vi "MEMR-Process Database.vi"() -> ()   [LabVIEW 2015]
uses:
  <vilib>/Analysis/NI_AALBase.lvlib
panel:
  out "Histogram Graph":T1(graph)={"X Values"=[-47.631112187359534, -42.893336562078595, -38.155560936797656, -33.41778531151672, -28.68000968623578, -23.942234060954842, -19.204458435673907, -14.466682810392967, -9.72890718511203, -4.991131559831092, -0.2533559345501544, 4.484419690730784, 9.222195316011721, 13.959970941292658, 18.697746566573596, 23.435522191854535, 28.17329781713547, 32.91107344241641, 37.64884906769735, 42.38662469297829], "Histogram: h(x)"=[2, 3, 2, 1, 2, 3, 5, 11, 7, 26, 28, 31, 12, 21, 13, 5, 5, 2, 1, 1]}
  in  "Analysis":T2={"Mode"=enum."at max gain", "T(ms) re peak"=2.0, "Fmin (Hz)"=800.0, "Fmax (Hz)"=3200.0, "Window"=enum."Hamming", "Resol (Hz)"=100.0, "Width (Hz)"=600.0, "Width (Hz) 2"=600.0}
  out "XY Graph":cluster{dbl[], dbl[]}[](graph)=[{[65.0, 70.0, 75.0, 70.0, 70.0, 65.0, 75.0, 70.0, 70.0, 70.0, 70.0, 70.0, 75.0, 85.0, 80.0, 80.0, 70.0, 75.0, 80.0, 80.0, 75.0, 65.0, 90.0, 90.0, 70.0, 75.0, 75.0, 65.0, 70.0, 70.0, 80.0, 75.0, 85.0, 80.0, 85.0, 80.0, 70.0, 65.0, 85.0, 80.0, 65.0, 75.0, 80.0, 75.0, 80.0, nan, 60.0, 60.0, 60.0, nan, 85.0, 80.0, 70.0, 70.0, 75.0, 85.0, 95.0, 75.0, 100.0, 85.0, 75.0, 90.0, 80.0, 75.0, 95.0, 90.0, 95.0, 90.0, 65.0, 75.0, nan, nan, 80.0, 80.0, 75.0, 90.0, 70.0, 85.0, 80.0, 50.0, 95.0, 90.0, 95.0, 85.0, 65.0, nan, 65.0, 75.0, 50.0, 65.0, 80.0, 80.0, 70.0, 90.0, 80.0, 70.0, 80.0, 75.0, 90.0, 85.0, 70.0, 70.0, 95.0, nan, 90.0, 80.0, 95.0, 100.0, 100.0, 100.0, 50.0, 85.0, 70.0, 50.0, 75.0, 75.0, 75.0, 75.0, 80.0, 85.0, 75.0, 75.0, 85.0, 70.0, 80.0, nan, 100.0, 85.0, 85.0, 80.0, 100.0, 75.0, 90.0, 85.0, 80.0, 75.0, 80.0, 75.0, 90.0, 90.0, 85.0, 75.0, 90.0, 90.0, 65.0, 85.0, 65.0, 65.0, 65.0, 85.0, 85.0, 90.0, nan, 85.0, 80.0, 75.0, 85.0, 80.0, 80.0, 75.0, 65.0, nan, 75.0, 70.0, 85.0, 75.0, 65.0, 75.0, 80.0, 75.0, 75.0, 50.0, 70.0, 80.0, 75.0, 70.0, 95.0, 85.0, 100.0, 90.0, 80.0, 80.0, 95.0, 90.0, 90.0, 50.0, 95.0, 95.0, 65.0, 75.0, 70.0, 70.0, 75.0, 80.0, 65.0, 65.0, 85.0, 60.0, 75.0, 70.0, 70.0, 75.0, 80.0, 80.0, 60.0, 85.0, 80.0, 75.0, 85.0, 80.0, 80.0, 80.0, 75.0, 75.0, nan, 80.0, 85.0, 80.0, 90.0, nan, 75.0, nan, 75.0, 80.0, 80.0, 70.0, nan, nan, 80.0, 50.0, 70.0, nan, 80.0, 70.0, 75.0, 60.0, 65.0, nan], [83.61038480664206, 88.90323491138284, nan, 76.6861342480343, 79.34245681049052, 66.14502666631483, 72.64039776246874, nan, 90.40140695048568, 73.59986593514996, 68.2285833975198, 68.95909577888109, 78.34029194041977, 66.40476363843403, nan, 88.4677553721679, 84.58576085004772, 62.13837967961564, 75.27817702322353, 71.94988571809287, 76.92571447237148, nan, 85.70082896210121, 87.89120704634068, 94.67191690824791, 79.80233146849612, 73.85409029034139, nan, 85.0, 93.55766432018085, 71.17769645171938, 85.4769276924145, nan, 84.75979569569505, 85.0, 85.52670684346738, 66.9788899682501, 69.20948606719492, 78.12781009882714, 79.19224304801239, 69.01017671276524, 67.64300936225919, 75.8043887454742, 73.85609821156797, 76.01253626857745, 85.0, 87.67149436103365, 66.75304409750719, 77.92784007393945, 82.44046631465581, 76.97482808652369, 78.44429598980619, 90.36011233515646, 57.49379196106444, 68.14676914537219, 78.66064680390217, nan, nan, nan, nan, 81.20509176100323, nan, 85.0, 70.33095954554724, 45.0, nan, 87.68722889473402, 85.25509994697506, 94.78893078630351, 77.75515257560767, 90.0, nan, nan, 94.8348417211292, 83.00419918222694, 93.18892634377539, 83.45013835841418, 72.03015940057925, 94.78202672029386, 79.7564120495189, 53.50224673653963, 85.84587239002288, 91.08548698295861, 46.25077363388457, 84.78546328663008, 91.01701177396114, 70.30568906673099, 78.99595778229026, 75.90995049601652, 85.02181316130722, 89.48615624550615, 81.1093912479705, 89.64413251768113, nan, 72.09675267675055, 81.72805574099463, 76.34503888270152, 75.67164645735843, 76.72561644593952, 54.108997651036915, 85.78378392899137, 78.47759249254159, 50.0, nan, nan, nan, 84.27014033057675, nan, 85.0, 89.83440652992289, 90.0, 63.3780833666432, 82.275627583266, 69.4041108088633, 77.55665508198922, 73.3088683958336, 86.90689069975696, 74.96703575207891, 82.37700129008836, 83.63890795813947, 72.19417062306756, 71.20730347534435, 90.95563139214721, 82.26302545197102, 59.757364077419076, 77.11292838155504, 87.08209177013414, nan, 80.0, 83.43169269612767, 53.73146823384199, 87.13006660761161, nan, 53.43379419404157, 80.01393285329306, 80.54156385472628, 80.21327744960064, 68.59887423802961, 70.0, nan, 82.77268093940407, 70.79201679725688, 88.65228346267106, 67.69603653315627, 70.0, 60.0, 90.0, 76.67991571420627, 80.0, 88.353883211932, 83.52892385361397, 70.0, 50.0, nan, 92.1153796896727, 77.80998882203835, nan, 89.76332680957675, 80.97331020337515, 72.83227440234356, 78.98506818754085, nan, 75.73931301525411, 85.0, 94.42464287719379, 84.08850701174643, nan, 75.35249373246242, 65.0, 90.0, 91.04866573115002, 80.90730659397525, 79.81740356491906, 85.0, 84.44661858514274, 90.48293650558534, 88.2586818731154, 77.00692996492972, nan, nan, 85.0, 83.56030129511086, 73.99166681322971, 75.0, 49.751203636703785, 43.722271947164565, 91.30805595730399, 65.0, nan, 75.09348869162191, 88.26860390703759, nan, 68.3141967304181, nan, 84.94480698741687, 87.85999618819487, 41.93345844004098, nan, nan, nan, nan, 90.0, 73.4554146040901, nan, 84.34738292000237, 68.43165488319733, 63.833644698525994, 91.47936652555856, 93.67058040834105, nan, nan, nan, 73.87445771753136, 78.30397650963862, 79.38295699025869, 93.49248113271616, 88.06829172475629, nan, nan, nan, 70.0, nan, 80.0, nan, 86.30759278580638, nan, 60.0, nan, 81.01066592260895, 94.75551250561875, nan, 91.62181131893622, 67.40528394856256, 72.50990150751193, 90.0, 94.1375552879297, 90.94631112233287, 74.72565053329737]}, ...(2 in all)]
  out "Progress":string="238/238"
  in  "Database":path=path "D:/Data/HHL/MEMR/database MEMR.csv"
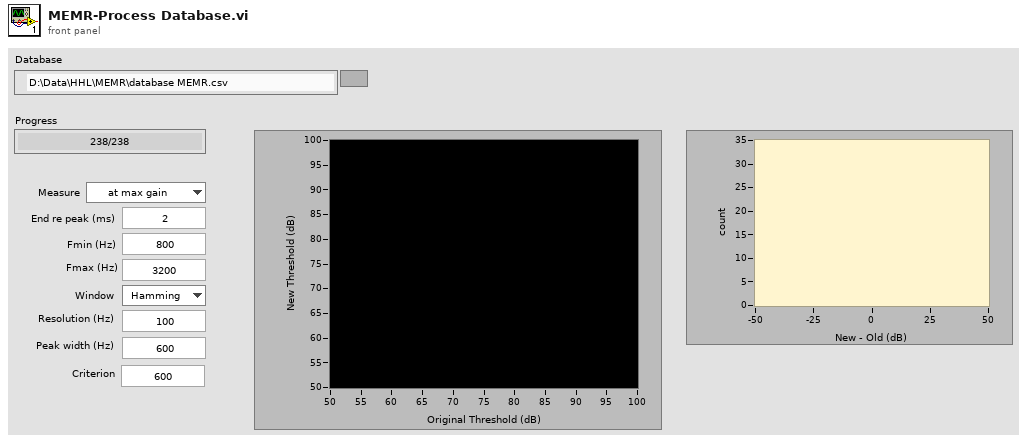
[diagram p1: front panel]
types:
  T1 = cluster{"X Values":dbl[], "Histogram: h(x)":i32[]}
  T2 = cluster{"Mode":enum16{"at max mag", "at max gain", "over window", "optimize"}, "T(ms) re peak":dbl, "Fmin (Hz)":dbl, "Fmax (Hz)":dbl, "Window":enum16{"None", "Hanning", "Hamming"}, "Resol (Hz)":dbl, "Width (Hz)":dbl, "Width (Hz) 2":dbl}
  T3 = enum16{"at max mag", "at max gain", "over window", "optimize"}
  T4 = cluster{"ID":i32, "Ear":string, "Run":i32[], "Original":dbl, "Paths":path[], "Threshold":dbl, "Strength":dbl}
  T5 = typedef "PDF-Catalog.ctl" = cluster{"report":refnum<class "PDF Report Class.lvclass">, "rows":i32, "cols":i32, "border":dbl, "width":dbl, "height":dbl, "next":i32}
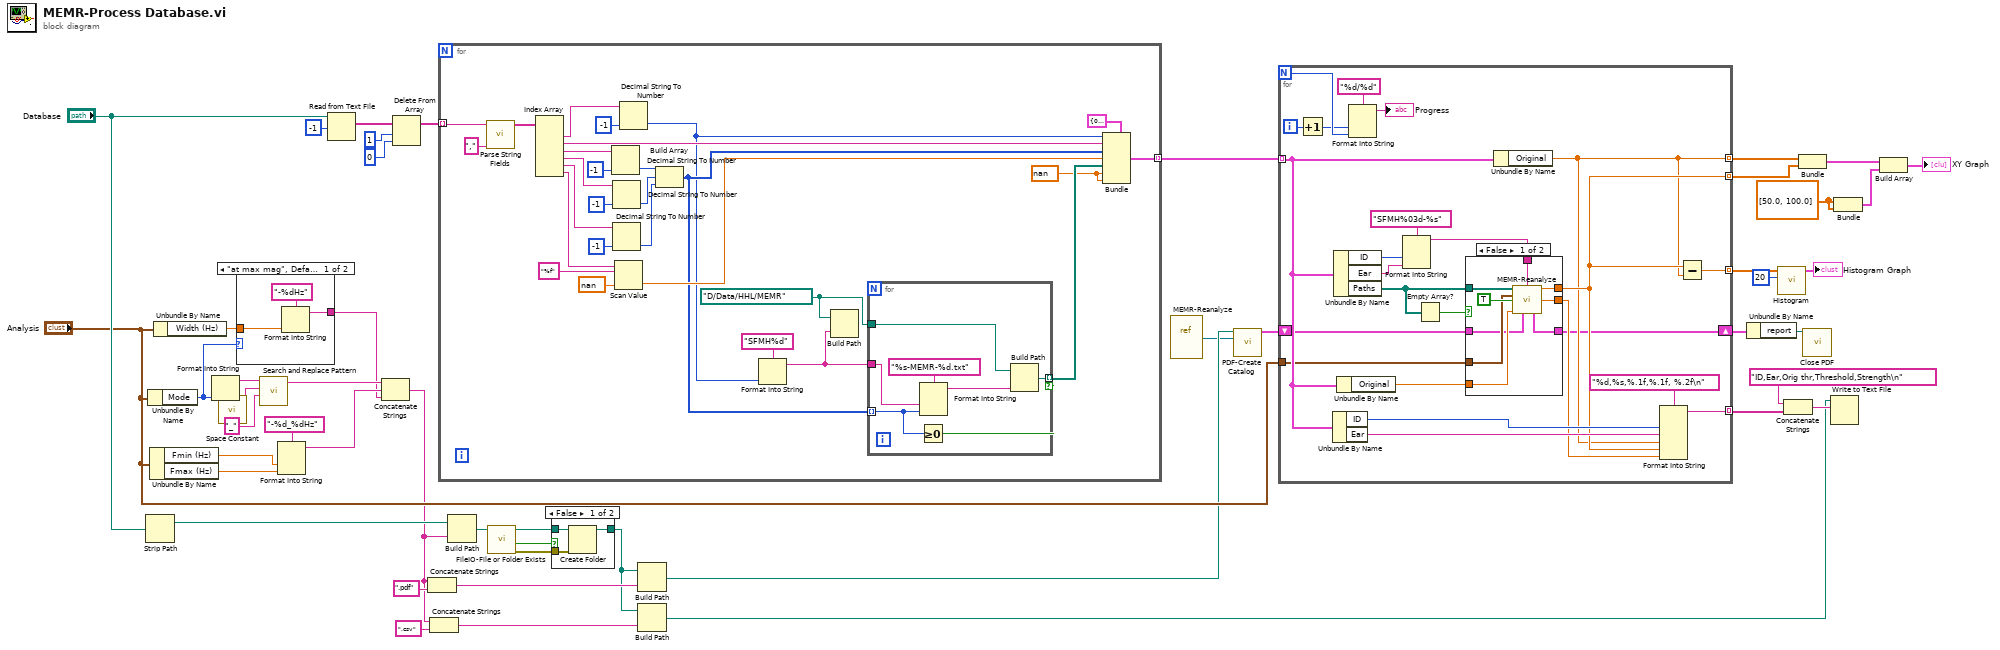
[diagram p0: block diagram]
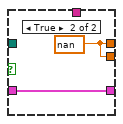
[diagram p4: hidden frame]
diagram:
  w40 = dbl[] [50.0, 100.0]
  n1 = Strip Path(path="Database") -> (stripped path=w19:path)  [unwired: 1 out]
  n2 = Unbundle By Name("Analysis") -> ("Mode"=w25:T3)
  n3 = Unbundle By Name("Analysis") -> ("Fmin (Hz)"=w27:dbl, "Fmax (Hz)"=w26:dbl)
  n4 = Unbundle By Name("Analysis") -> ("Width (Hz)"=w23:dbl)
  n5 = Format Into String(w25) -> (resulting string=w31:string)  [unwired: 3 in, 1 out]
  n6 = call <vilib>:"Space Constant.vi"() -> ("String"=w30:string)
  n7 = case shown="\"at max mag\", Default" w25 {
    tunnel: w23 -> [w51 _]
    tunnel: [w49 _] -> w20
    frame "at max mag", Default {
      n8 = Format Into String(format string="-%dHz", w51) -> (resulting string=w49:string)  [unwired: 2 in, 1 out]
    }
    frame "over window" {
    }
  }
  n9 = call <vilib>:"Search and Replace Pattern.vi"("string"=w31, "regular expression (\"\")"=w30, "replace string (\"\")"="_" ("replace string (\"\")")) -> ("result string"=w22:string)  [unwired: 2 in, 1 out]
  n10 = Format Into String(format string="-%d_%dHz", w27, w26) -> (resulting string=w21:string)  [unwired: 2 in, 1 out]
  n11 = Read from Text File(file (use dialog)="Database", count=-1) -> (text=w47:string[])  [unwired: 2 in, 3 out]
  n12 = Concatenate Strings(w22, w21, w20) -> (w7:string)
  n13 = Delete From Array(array=w47, length=1, index=0) -> (array with subset deleted=w44:string[])  [unwired: 1 out]
  n14 = Concatenate Strings(w7, ".pdf" ("string")) -> (w9:string)
  n15 = Concatenate Strings(w7, ".csv" ("string")) -> (w17:string)
  n16 = for {
    tunnel: w44 -> [w79] mode=indexing
    tunnel: [w63] -> w37 mode=indexing
    w53 = nan
    w52 = path "D:/Data/HHL/MEMR"
    n17 = call "Parse String Fields.vi"("Separator"=",", "String"=w79) -> ("Fields"=w77:string[])  [unwired: 8 in, 1 out]
    n18 = Index Array(array=w77) -> (element #1=w55:string, element #2=w58:string, element #3=w76:string, element #4=w72:string, element #5=w71:string, element #6=w70:string)  [unwired: 6 in]
    n19 = Decimal String To Number(string=w76, default (0L)=-1 ("default (0 I32)")) -> (number=w67:i32)  [unwired: 1 in, 1 out]
    n20 = Decimal String To Number(string=w72, default (0L)=-1 ("default (0 I32)")) -> (number=w66:i32)  [unwired: 1 in, 1 out]
    n21 = Decimal String To Number(string=w71, default (0L)=-1 ("default (0 I32)")) -> (number=w65:i32)  [unwired: 1 in, 1 out]
    n22 = Scan Value(string=w70, format string="%f", default (0 dbl)=nan) -> (value=w64:dbl)  [unwired: 1 out]
    n23 = Decimal String To Number(string=w55, default (0L)=-1 ("default (0 I32)")) -> (number=w54:i32)  [unwired: 1 in, 1 out]
    n24 = Build Array(w67, w66, w65) -> (w59:i32[])
    n25 = Format Into String(format string="SFMH%d", w54) -> (resulting string=w60:string)  [unwired: 2 in, 1 out]
    n26 = Build Path(base path=w52, name or relative path=w60) -> ()  [unwired: 1 out]
    n27 = for {
      tunnel: w52 -> [w83]
      tunnel: w59 -> [w81] mode=indexing
      tunnel: w60 -> [w85]
      tunnel: [w82] -> w57 mode=indexing if=w80
      n28 = Greater Or Equal To 0?(x=w81) -> (x >= 0?=w80:bool)
      n29 = Format Into String(format string="%s-MEMR-%d.txt", w85, w81) -> (resulting string=w84:string)  [unwired: 2 in, 1 out]
      n30 = Build Path(base path=w83, name or relative path=w84) -> (appended path=w82:path)
    }
    n31 = Bundle(cluster=T4 {"ID"=0, "Ear"="R", "Run"=[19, 20, 21], "Original"=65.0, "Paths"=[], "Threshold"=65.0, "Strength"=nan}, "ID"=w54, "Ear"=w58, "Run"=w59, "Original"=w64, "Paths"=w57, "Threshold"=w53, "Strength"=w53) -> (w63:T4)
  }
  n32 = Build Path(base path=w19, name or relative path=w7) -> (appended path=w8:path)
  n33 = call "FileIO-File or Folder Exists.vi"("path"=w8) -> ("error out"=w13:errorcluster, "Exists?"=w11:bool, "dup path"=w12:path)  [unwired: 7 in, 1 out]
  n34 = case shown="False" w11 {
    tunnel: [w89 w90] -> w3
    tunnel: w13 -> [w88 _]
    tunnel: w12 -> [w87 w90]
    frame False {
      n35 = Create Folder(path (use dialog)=w87, error in=w88) -> (created path=w89:path)  [unwired: 1 in, 2 out]
    }
    frame True {
    }
  }
  n36 = Build Path(base path=w3, name or relative path=w9) -> (appended path=w6:path)
  n37 = Build Path(base path=w3, name or relative path=w17) -> (appended path=w14:path)
  n38 = vi-ref "MEMR-Reanalyze.vi"() -> (w1:refnum<vi>)
  n39 = call "PDF-Create Catalog.vi"("PDF Path"=w6, "VI"=w1) -> ("catalog"=w5:T5)  [unwired: 12 in, 1 out]
  n40 = for {
    N -> [w109]
    tunnel: w37 -> [w102] mode=indexing
    tunnel: [w95] -> w43 mode=indexing
    tunnel: [w96] -> w42 mode=indexing
    tunnel: [w98] -> w36 mode=indexing
    tunnel: [w97] -> w35 mode=indexing
    tunnel: "Analysis" -> [w94]
    shift-right: [w92] -> w4
    shift-left: w5 -> [w93]
    i -> [w110]
    n41 = Increment(x=w110) -> (x+1=w107:i32)
    n42 = Unbundle By Name(w102) -> ("ID"=w101:i32, "Ear"=w100:string)
    n43 = Unbundle By Name(w102) -> ("ID"=w113:i32, "Ear"=w112:string, "Paths"=w106:path[])
    n44 = Unbundle By Name(w102) -> ("Original"=w104:dbl)
    n45 = Format Into String(format string="%d/%d", w107, w109) -> (resulting string=→"Progress":string)  [unwired: 2 in, 1 out]
    n46 = Format Into String(format string="SFMH%03d-%s", w113, w112) -> (resulting string=w91:string)  [unwired: 2 in, 1 out]
    n47 = Empty Array?(array=w106) -> (empty?=w105:bool)
    n48 = case shown="False" w105 {
      tunnel: [w122 w125] -> w96
      tunnel: w106 -> [w121 _]
      tunnel: w104 -> [w120 _]
      tunnel: [w119 w125] -> w99
      tunnel: w94 -> [w118 _]
      tunnel: w93 -> [w117 w124]
      tunnel: [w116 w124] -> w92
      tunnel: w91 -> [w115 _]
      frame False {
        n49 = call "MEMR-Reanalyze.vi"("Path"=w121, "Caption"=w115, "Threshold"=w118, "Plot?"=TRUE, "Original"=w120, "catalog in"=w117) -> ("Threshold"=w122:dbl, "Strength"=w119:dbl, "catalog out"=w116:T5)  [unwired: 7 in]
      }
      frame True {
        w125 = nan ("Threshold")
      }
    }
    n50 = Unbundle By Name(w102) -> ("Original"=w95:dbl)
    n51 = Format Into String(format string="%d,%s,%.1f,%.1f, %.2f\n", w101, w100, w95, w96, w99) -> (resulting string=w98:string)  [unwired: 2 in, 1 out]
    n52 = Subtract(x=w96, y=w95) -> (x-y=w97:dbl)
  }
  n53 = Unbundle By Name(w4) -> ("report"=w2:refnum<class "PDF Report Class.lvclass">)
  n54 = call <vilib>:"Histogram.vi"("intervals"=20, "X"=w35) -> ("Histogram Graph"=→"Histogram Graph":T1)  [unwired: 6 in, 3 out]
  n55 = Concatenate Strings("ID,Ear,Orig thr,Threshold,Strength\n" ("format string"), w36) -> (w15:string)
  n56 = Bundle(w43, w42) -> (w41:cluster{dbl[], dbl[]})  [unwired: 1 in]
  n57 = call <vilib>:"Close PDF.vi"("PDF Report"=w2) -> ()  [unwired: 13 in, 2 out]
  n58 = Write to Text File(file (use dialog)=w14, text=w15) -> ()  [unwired: 2 in, 3 out]
  n59 = Bundle(w40, w40) -> (w38:cluster{dbl[], dbl[]})  [unwired: 1 in]
  n60 = Build Array(w41, w38) -> (→"XY Graph":cluster{dbl[], dbl[]}[])
